vi "Load Test.vi"(8 "error in (no error)":errorcluster, 10 "Test Result 2":refnum<vi>, 11 "Data In":T1={"Message"="", "Homed?"=FALSE, "NextState"=enum."Timeout", "G.Load"=0.0, "G.Position"=0.0, "Load#"=0, "[G.Loads]"=[], "[TotalLoads]"=[], "[Errors]"=[], "ZeroWait"=0, "Results"=[], "DwellWait"=FALSE, "Test Result"=FALSE, "[CondyleLoads]"=[], "[Max]"=[], "[Min]"=[], "Valid String?"=FALSE, "ScanTime"=timestamp(0 s since 1904-01-01), "ScannedString"="", "LabelDevID"=0, "MfgDate"=timestamp(0 s since 1904-01-01), "[EEPROM Cmds]"=[], "[CalData]"=[], "[A/Ds]"=[], "[A/Dmax]"=[], "[A/Dmin]"=[], "BattMax"=0.0, "BattMin"=0.0, "DwellTime"=2000, "PendingDeviceType"="", "Zero G.load"=0.0, "GAINC Value"="", "Programming Step"=enum."Load EEPROM", "Front Panel Program?"=FALSE, "Final Program?"=FALSE, "PCB Score"=100, "AssyScore"=100, "Pass/Fail #"="", "Result String"="", "Programming Mode"=enum."Initial Program", "Angle Test Step"=enum."Initialize", "Accel Values"=[], "Shutdown Counter"=0, "V1"=0, "V2"=0, "V3"=0, "V4"=0, "EEPROM Data"=[], "Counter"=0, "Page#"=0, "Timer"=timestamp(0 s since 1904-01-01), "Use Mark10?"=FALSE, "Eng-Result#"=0, "DUT Serial #"=0, "Scroll Message?"=FALSE, "Clear Message"=FALSE, "Batt Test Step "=enum."Initialize", "RXTX Window Found?"=FALSE, "Shutdown First Call?"=FALSE, "A2 Delay (msec)"=500, "Support Script"={"Script #"="", "Script Revision"="", "[OEMs]"=[], "[[DeviceTypes]]"=[], "[[DeviceTypesVals]]"=[], "[[List of Errors]]"=[], "Default GAINC"="", "[[ASICtrims]]"=[], "ID For Echo"="", "Condyle A CalFactor"=100, "Condyle B CalFactor"=100, "[OEMs Prefix]"=[], "Packet ID 18"="", "[[Force Table Load Test]]"=[], "[[Force Table AccurTest]]"=[]}, "Serial Table"={"Serial File Path"=path "", "[[Serial Lookup Table]]"=[], "Serial Device Info"=[], "Valid Serial?"=FALSE}, "Target Information"={"Target Brand"="", "Target DeviceType"="", "Target Serial#"=100, "Target Lot#"=0, "Target DevID"=0, "Target Channel"=5}, "Operator"="", "COM Port"="", "Config Path"=path "", "Tx Array"=[], "DUT Parameters"={"Channel"=0, "DeviceID"=0, "Script Rev"=0, "Month"=0, "Day"=0, "Year"=0, "Lot#"=0, "V1"=0, "V2"=0, "V3"=0, "V4"=0, "MFG"=0, "Cal FactorA 10"=0, "Cal FactorB 10  "=0, "Cal FactorA 16"=0, "Cal FactorB 16"=0, "ASICtrim"=[], "TmpChan"=0, "GAINC"="", "Brand"="", "Device"="", "Serial #"=0, "Batt310"=0, "Batt 280"=0}, "FTS Main?"=FALSE, "Loading"={"[Forces]"=[], "[Dwell]"=[], "Loading Step"=enum."Initialize Test"}, "Software Version"="", "Correction Factor"="", "Second Load Test"=FALSE, "Acc Loads"=[], "Mark10 Config"={"H2S%"=[80.0, 85.0, 90.0, 95.0, 100.0], "H2S Speed"=[12.0, 8.0, 6.0, 4.0, 2.0], "H to S"=2.0, "Home Speed"=1.0, "LoadWin"=0.0, "Load Speed"=0.0, "PID"={"Kp"=0.04, "Kd"=0.005001, "Ki"=2.9999999999999923e-05}}, "Channels"={"Transceiver Ch"=5, "Operating Ch"=5, "Start Ch"=0}, "Channel EEPROM"=[], "Load Notes"=[], "Engr Log?"=FALSE, "Time"=[], "Program Retry"=FALSE, "Operator Channel"="", "Target Channel "="", "New Data Program"=FALSE, "NFHU Pass?"=FALSE, "Cycle Number"=0, "Cal Cycle#"=0, "[Avg G.Loads] "=[], "[Avg A/Ds] "=[], "Cal Retry?"=FALSE, "[Total A/Ds]  "=[], "Cycle Num LA"=0, "LA Cycle# "=0, "Shim Num"=0, "Shim#  "=0, "Angle Test?"=FALSE} {"Mark10 Config"."PID"."Ki" min=0.0 max=200.0 format="%.6f"; "Mark10 Config"."PID"."Kd" min=0.0 max=200.0 format="%.6f"; "Mark10 Config"."PID"."Kp" min=0.0 max=200.0 format="%.6f"; "DUT Parameters"."ASICtrim" format="%02x"}) -> (0 "error out":errorcluster, 1 "LoadSensors":dbl[](array[numeric]), 3 "State-machine Local Variables out":T1={"Message"="", "Homed?"=FALSE, "NextState"=enum."Timeout", "G.Load"=0.0, "G.Position"=0.0, "Load#"=0, "[G.Loads]"=[], "[TotalLoads]"=[], "[Errors]"=[], "ZeroWait"=0, "Results"=[], "DwellWait"=FALSE, "Test Result"=FALSE, "[CondyleLoads]"=[], "[Max]"=[], "[Min]"=[], "Valid String?"=FALSE, "ScanTime"=timestamp(0 s since 1904-01-01), "ScannedString"="", "LabelDevID"=0, "MfgDate"=timestamp(0 s since 1904-01-01), "[EEPROM Cmds]"=[], "[CalData]"=[], "[A/Ds]"=[], "[A/Dmax]"=[], "[A/Dmin]"=[], "BattMax"=0.0, "BattMin"=0.0, "DwellTime"=2000, "PendingDeviceType"="", "Zero G.load"=0.0, "GAINC Value"="", "Programming Step"=enum."Load EEPROM", "Front Panel Program?"=FALSE, "Final Program?"=FALSE, "PCB Score"=100, "AssyScore"=100, "Pass/Fail #"="", "Result String"="", "Programming Mode"=enum."Initial Program", "Angle Test Step"=enum."Initialize", "Accel Values"=[], "Shutdown Counter"=0, "V1"=0, "V2"=0, "V3"=0, "V4"=0, "EEPROM Data"=[], "Counter"=0, "Page#"=0, "Timer"=timestamp(0 s since 1904-01-01), "Use Mark10?"=FALSE, "Eng-Result#"=0, "DUT Serial #"=0, "Scroll Message?"=FALSE, "Clear Message"=FALSE, "Batt Test Step "=enum."Initialize", "RXTX Window Found?"=FALSE, "Shutdown First Call?"=FALSE, "A2 Delay (msec)"=500, "Support Script"={"Script #"="", "Script Revision"="", "[OEMs]"=[], "[[DeviceTypes]]"=[], "[[DeviceTypesVals]]"=[], "[[List of Errors]]"=[], "Default GAINC"="", "[[ASICtrims]]"=[], "ID For Echo"="", "Condyle A CalFactor"=100, "Condyle B CalFactor"=100, "[OEMs Prefix]"=[], "Packet ID 18"="", "[[Force Table Load Test]]"=[], "[[Force Table AccurTest]]"=[]}, "Serial Table"={"Serial File Path"=path "", "[[Serial Lookup Table]]"=[], "Serial Device Info"=[], "Valid Serial?"=FALSE}, "Target Information"={"Target Brand"="", "Target DeviceType"="", "Target Serial#"=100, "Target Lot#"=0, "Target DevID"=0, "Target Channel"=5}, "Operator"="", "COM Port"="", "Config Path"=path "", "Tx Array"=[], "DUT Parameters"={"Channel"=0, "DeviceID"=0, "Script Rev"=0, "Month"=0, "Day"=0, "Year"=0, "Lot#"=0, "V1"=0, "V2"=0, "V3"=0, "V4"=0, "MFG"=0, "Cal FactorA 10"=0, "Cal FactorB 10  "=0, "Cal FactorA 16"=0, "Cal FactorB 16"=0, "ASICtrim"=[], "TmpChan"=0, "GAINC"="", "Brand"="", "Device"="", "Serial #"=0, "Batt310"=0, "Batt 280"=0}, "FTS Main?"=FALSE, "Loading"={"[Forces]"=[], "[Dwell]"=[], "Loading Step"=enum."Initialize Test"}, "Software Version"="", "Correction Factor"="", "Second Load Test"=FALSE, "Acc Loads"=[], "Mark10 Config"={"H2S%"=[80.0, 85.0, 90.0, 95.0, 100.0], "H2S Speed"=[12.0, 8.0, 6.0, 4.0, 2.0], "H to S"=2.0, "Home Speed"=1.0, "LoadWin"=0.0, "Load Speed"=0.0, "PID"={"Kp"=0.04, "Kd"=0.005001, "Ki"=2.9999999999999923e-05}}, "Channels"={"Transceiver Ch"=5, "Operating Ch"=5, "Start Ch"=0}, "Channel EEPROM"=[], "Load Notes"=[], "Engr Log?"=FALSE, "Time"=[], "Program Retry"=FALSE, "Operator Channel"="", "Target Channel "="", "New Data Program"=FALSE, "NFHU Pass?"=FALSE, "Cycle Number"=0, "Cal Cycle#"=0, "[Avg G.Loads] "=[], "[Avg A/Ds] "=[], "Cal Retry?"=FALSE, "[Total A/Ds]  "=[], "Cycle Num LA"=0, "LA Cycle# "=0, "Shim Num"=0, "Shim#  "=0, "Angle Test?"=FALSE} {"Mark10 Config"."PID"."Ki" min=0.0 max=200.0 format="%.6f"; "Mark10 Config"."PID"."Kd" min=0.0 max=200.0 format="%.6f"; "Mark10 Config"."PID"."Kp" min=0.0 max=200.0 format="%.6f"; "DUT Parameters"."ASICtrim" format="%02x"}, 5 "Raw Data":u16[](array[numeric]))   [LabVIEW 2015]
uses:
  Controls/LocalVars.ctl
  Controls/Gen2 FT states.ctl
  Controls/Iniial Device Programming.ctl
  ProgramStageControl.ctl
  Controls/Batt Cap Steps.ctl
  Controls/Support Script.ctl
  Controls/Serial Table.ctl
  Controls/Device Information.ctl
  Controls/InfoPacket.ctl
  Controls/Loading.ctl
  Controls/Load Step.ctl
  Controls/Mark10 Config.ctl
  Controls/PID parameters.ctl
  Controls/Channels.ctl
  Controls/Mark10 states.ctl
  Controls/Gen2 FT Globals.vi
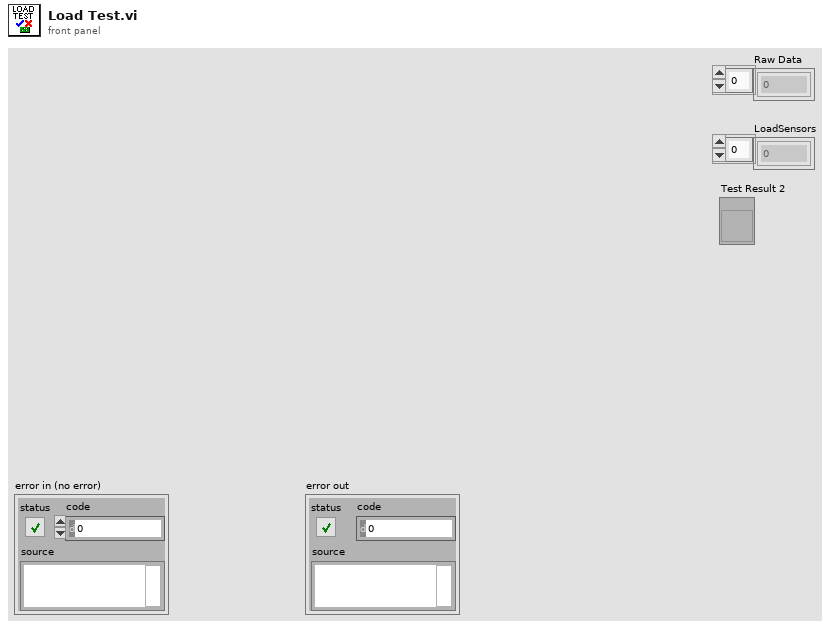
[diagram p1: front panel]
types:
  T1 = typedef "LocalVars.ctl" = cluster{"Message":string, "Homed?":bool, "NextState":T2, "G.Load":dbl, "G.Position":dbl, "Load#":i32, "[G.Loads]":dbl[], "[TotalLoads]":dbl[], "[Errors]":dbl[][], "ZeroWait":u32, "Results":dbl[], "DwellWait":bool, "Test Result":bool, "[CondyleLoads]":dbl[][], "[Max]":dbl[], "[Min]":dbl[], "Valid String?":bool, "ScanTime":timestamp, "ScannedString":string, "LabelDevID":u32, "MfgDate":timestamp, "[EEPROM Cmds]":u8[][], "[CalData]":u8[][], "[A/Ds]":dbl[][], "[A/Dmax]":dbl[], "[A/Dmin]":dbl[], "BattMax":dbl, "BattMin":dbl, "DwellTime":i32, "PendingDeviceType":string, "Zero G.load":dbl, "GAINC Value":string, "Programming Step":T3, "Front Panel Program?":bool, "Final Program?":bool, "PCB Score":i32, "AssyScore":i32, "Pass/Fail #":string, "Result String":string, "Programming Mode":T4, "Angle Test Step":enum16{"Initialize", "Get X", "Get Y", "Get Z", "Next Test"}, "Accel Values":dbl[][], "Shutdown Counter":u32, "V1":i32, "V2":i32, "V3":i32, "V4":i32, "EEPROM Data":i32[][], "Counter":i32, "Page#":i32, "Timer":timestamp, "Use Mark10?":bool, "Eng-Result#":u32, "DUT Serial #":i32, "Scroll Message?":bool, "Clear Message":bool, "Batt Test Step ":T5, "RXTX Window Found?":bool, "Shutdown First Call?":bool, "A2 Delay (msec)":i16, "Support Script":T6, "Serial Table":T7, "Target Information":T8, "Operator":string, "COM Port":string, "Config Path":path, "Tx Array":u8[], "DUT Parameters":T9, "FTS Main?":bool, "Loading":T10, "Software Version":string, "Correction Factor":string, "Second Load Test":bool, "Acc Loads":dbl[][], "Mark10 Config":T12, "Channels":T14, "Channel EEPROM":i32[][], "Load Notes":string[], "Engr Log?":bool, "Time":timestamp[], "Program Retry":bool, "Operator Channel":string, "Target Channel ":string, "New Data Program":bool, "NFHU Pass?":bool, "Cycle Number":i32, "Cal Cycle#":i32, "[Avg G.Loads] ":dbl[], "[Avg A/Ds] ":dbl[][], "Cal Retry?":bool, "[Total A/Ds]  ":dbl[][], "Cycle Num LA":i32, "LA Cycle# ":i32, "Shim Num":i32, "Shim#  ":i32, "Angle Test?":bool}
  T2 = typedef "Gen2 FT states.ctl" = enum16{"---------SETUP-------", "Initialization", "Read Support Data", "Initialize Mark-10", "Initialize Transceiver", "------UTILITIES------", "Change DUT Channel", "Find RxTx Window", "Reset Device", "Scan Channels", "Read Serial Lookup", "Shutdown Device", "ESTOP", "--------USER---------", "Timeout", "-----PROGRAM-----", "Program Device", "------MARK10--------", "Go Home", "MoveUp", "MoveDown", "Goto Load", "Goto Position", "Stop Motor", "---------TESTS--------", "Start Test", "Angle Test", "Load Test", "Load Accuracy Test", "Battery Test", "------RESULTS-------", "End Test", "Display Result", "--------EXIT--------", "Exit"}
  T3 = typedef "Iniial Device Programming.ctl" = enum16{"Load EEPROM", "Send First A1", "Send EEPROM", "Send A1", "Check EEPROM Echo", "Verify transmission", "Programming Successful", "Programming Failed"}
  T4 = typedef "ProgramStageControl.ctl" = enum16{"Initial Program", "GainC", "Scales"}
  T5 = typedef "Batt Cap Steps.ctl" = enum16{"Initialize", "Collect 2.8 Volts", "Collect 3.1 Volts", "Check Results"}
  T6 = typedef "Support Script.ctl" = cluster{"Script #":string, "Script Revision":string, "[OEMs]":string[], "[[DeviceTypes]]":string[][], "[[DeviceTypesVals]]":u16[][], "[[List of Errors]]":string[][], "Default GAINC":string, "[[ASICtrims]]":u8[][], "ID For Echo":string, "Condyle A CalFactor":i32, "Condyle B CalFactor":i32, "[OEMs Prefix]":string[], "Packet ID 18":string, "[[Force Table Load Test]]":dbl[][], "[[Force Table AccurTest]]":dbl[][]}
  T7 = typedef "Serial Table.ctl" = cluster{"Serial File Path":path, "[[Serial Lookup Table]]":string[][], "Serial Device Info":string[], "Valid Serial?":bool}
  T8 = typedef "Device Information.ctl" = cluster{"Target Brand":string, "Target DeviceType":string, "Target Serial#":i32, "Target Lot#":u32, "Target DevID":u32, "Target Channel":u8}
  T9 = typedef "InfoPacket.ctl" = cluster{"Channel":u8, "DeviceID":u32, "Script Rev":u8, "Month":u8, "Day":u8, "Year":u8, "Lot#":u32, "V1":u16, "V2":u16, "V3":u16, "V4":u16, "MFG":u8, "Cal FactorA 10":u8, "Cal FactorB 10  ":u8, "Cal FactorA 16":u8, "Cal FactorB 16":u8, "ASICtrim":u8[], "TmpChan":u8, "GAINC":string, "Brand":string, "Device":string, "Serial #":u64, "Batt310":u16, "Batt 280":u16}
  T10 = typedef "Loading.ctl" = cluster{"[Forces]":dbl[], "[Dwell]":dbl[], "Loading Step":T11}
  T11 = typedef "Load Step.ctl" = enum16{"Initialize Test", "Go Home", "Detect Dev Surface", "Wait to zero Device", "Zero Device", "Do Test", "Test Result"}
  T12 = typedef "Mark10 Config.ctl" = cluster{"H2S%":dbl[], "H2S Speed":dbl[], "H to S":dbl, "Home Speed":dbl, "LoadWin":dbl, "Load Speed":dbl, "PID":T13}
  T13 = typedef "PID parameters.ctl" = cluster{"Kp":dbl, "Kd":dbl, "Ki":dbl}
  T14 = typedef "Channels.ctl" = cluster{"Transceiver Ch":u8, "Operating Ch":u8, "Start Ch":u8}
  T15 = typedef "DeviceInfo.ctl" = cluster{"DevInfo":T9, "Mfg Date":timestamp, "[CalData]":u8[][], "[DevData]":u8[], "GotCal":bool, "CustomCal?":bool, "Packet#":i32}
  T16 = typedef "Mark10 states.ctl" = enum16{"Initialize", "Go Home", "Move Up", "Move Down", "Stop @ Load", "Read Status", "Goto Position", "Goto Device Surface", "Stop Motor", "Shutdown", "Exit"}
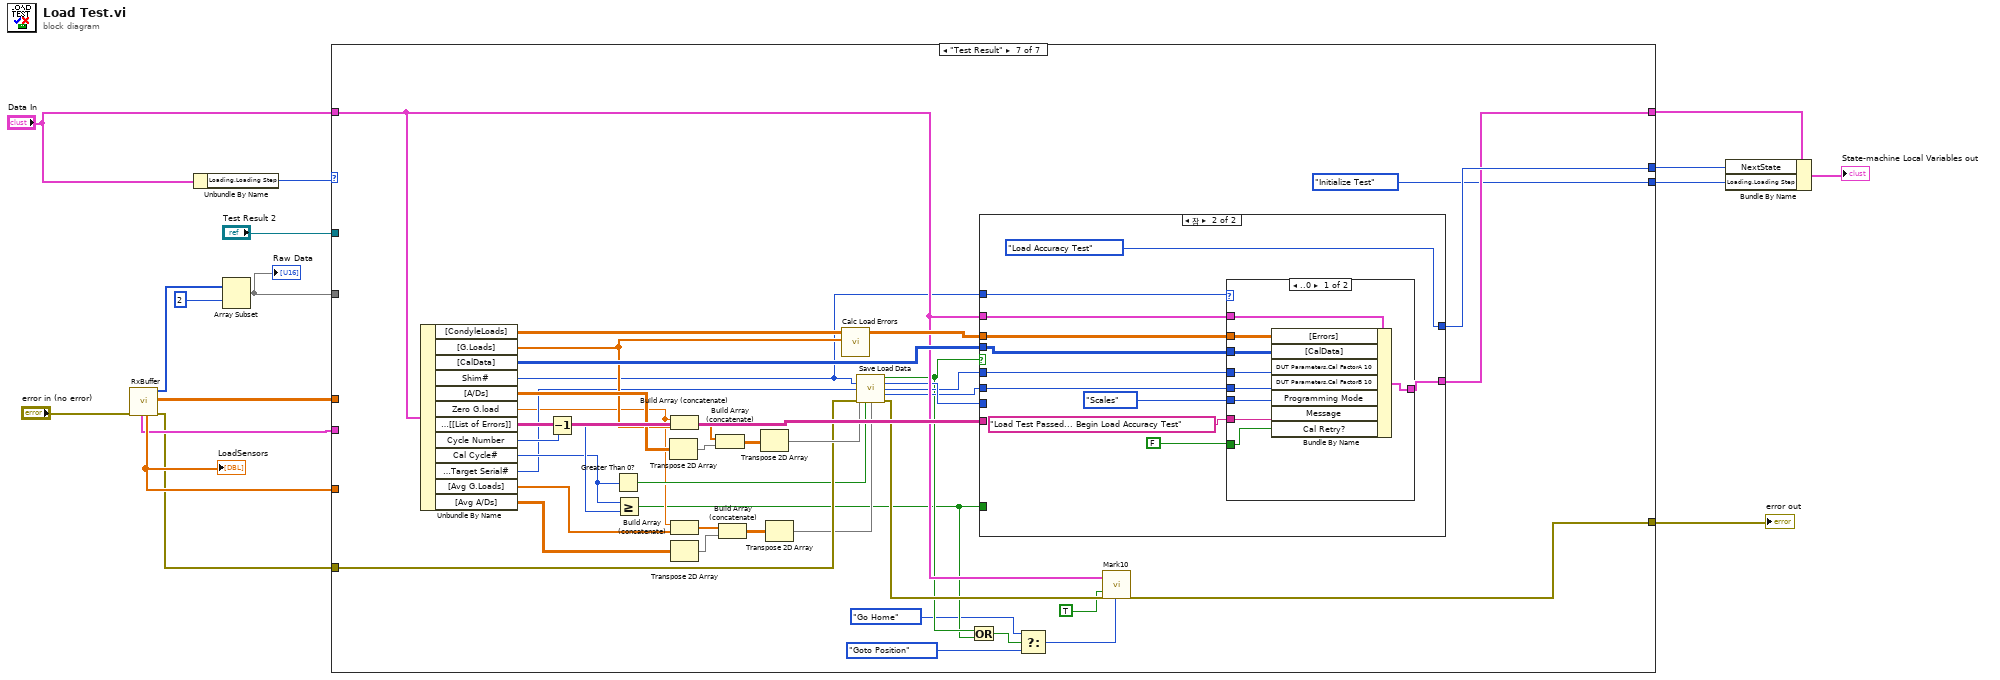
[diagram p0: block diagram]
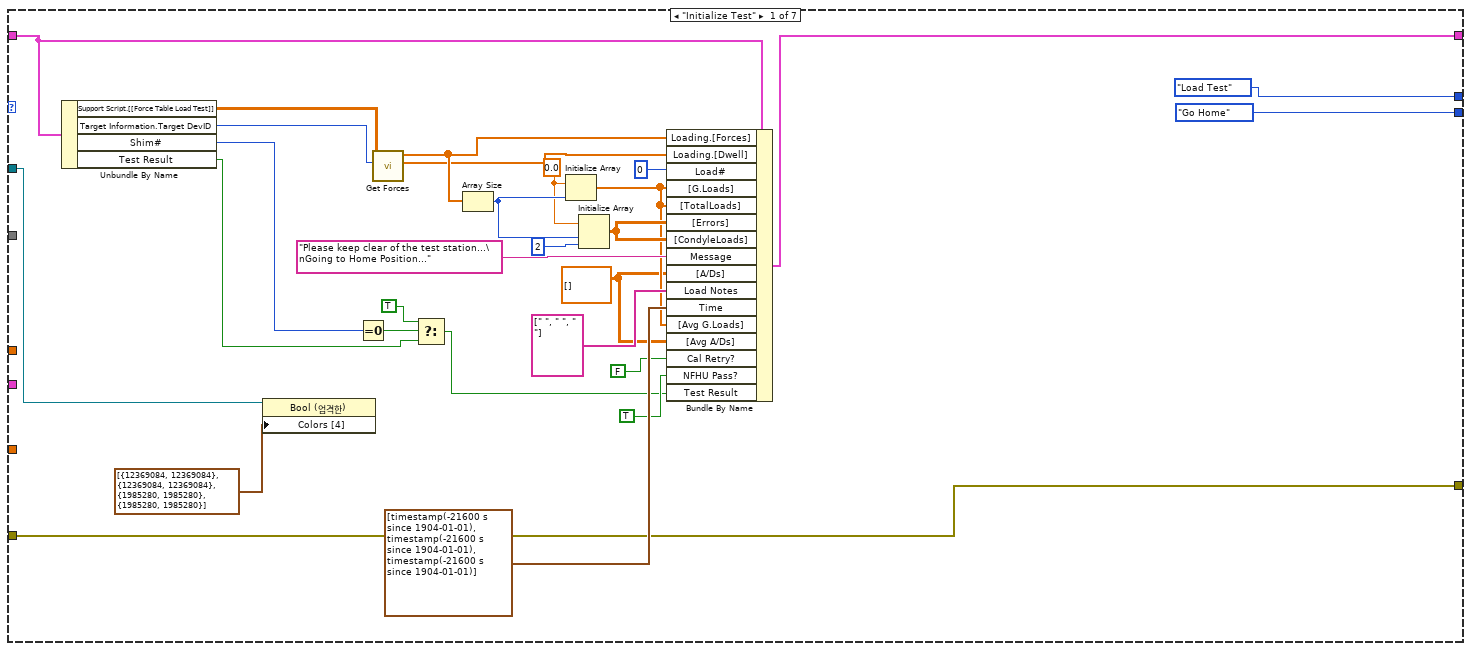
[diagram p2: hidden frame]
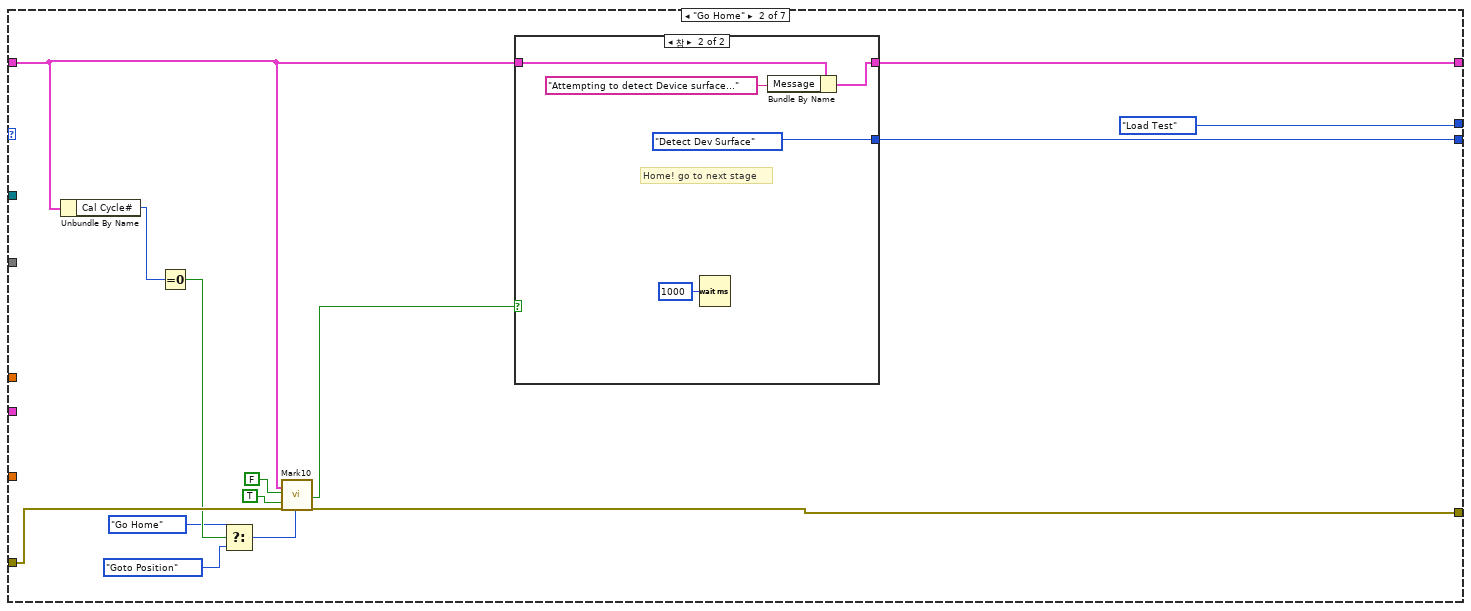
[diagram p3: hidden frame]
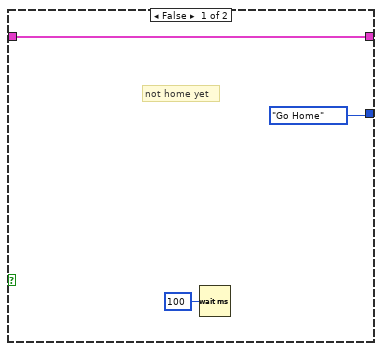
[diagram p4: hidden frame]
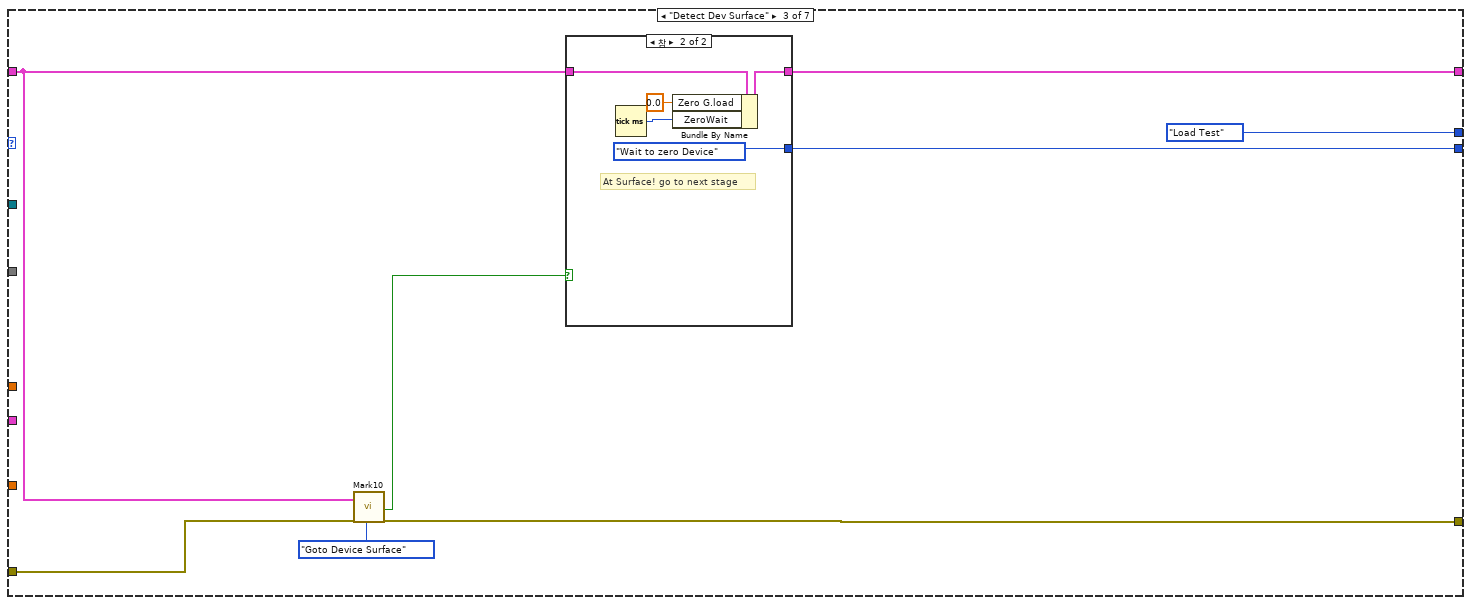
[diagram p5: hidden frame]
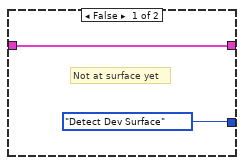
[diagram p6: hidden frame]
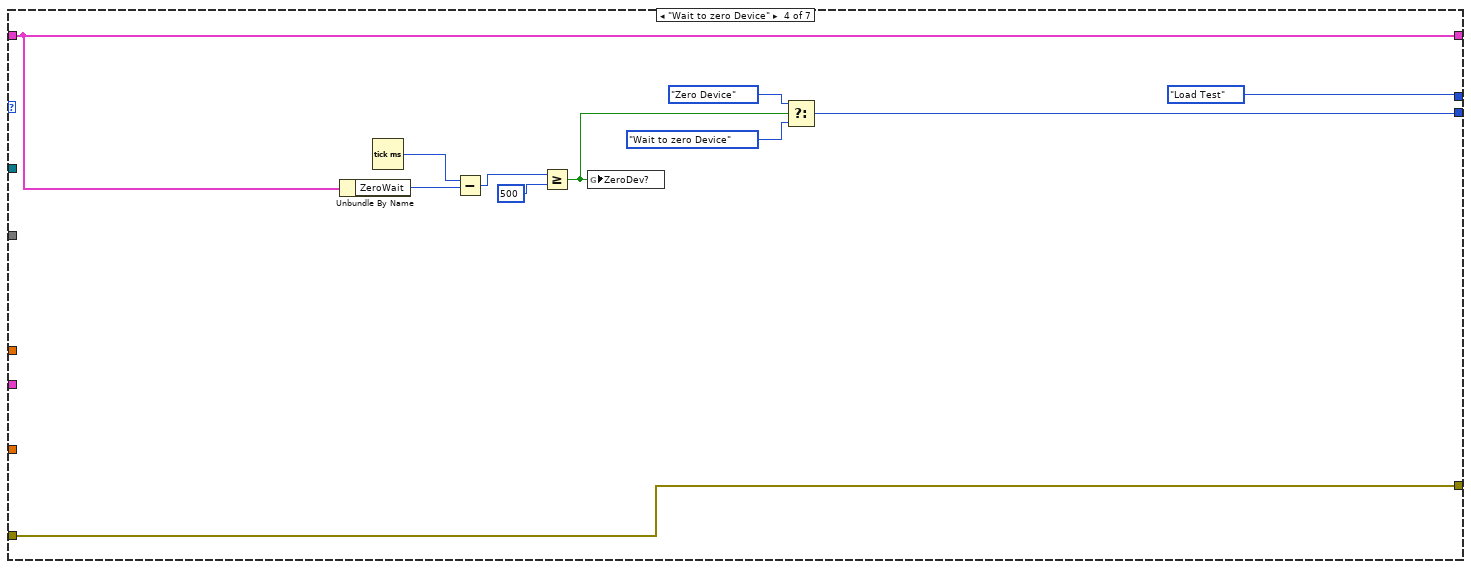
[diagram p7: hidden frame]
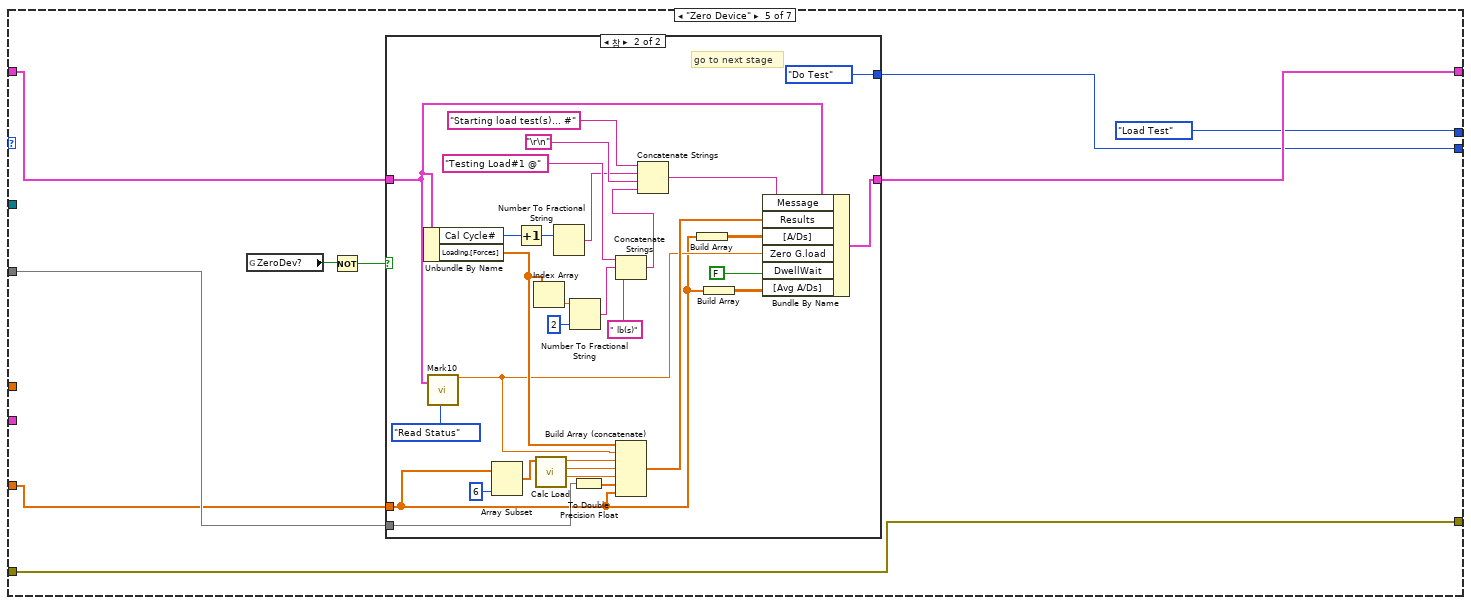
[diagram p8: hidden frame]
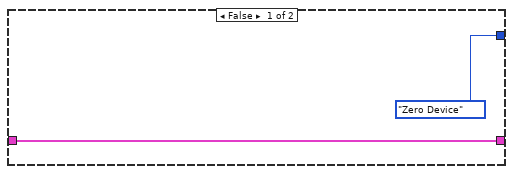
[diagram p9: hidden frame]
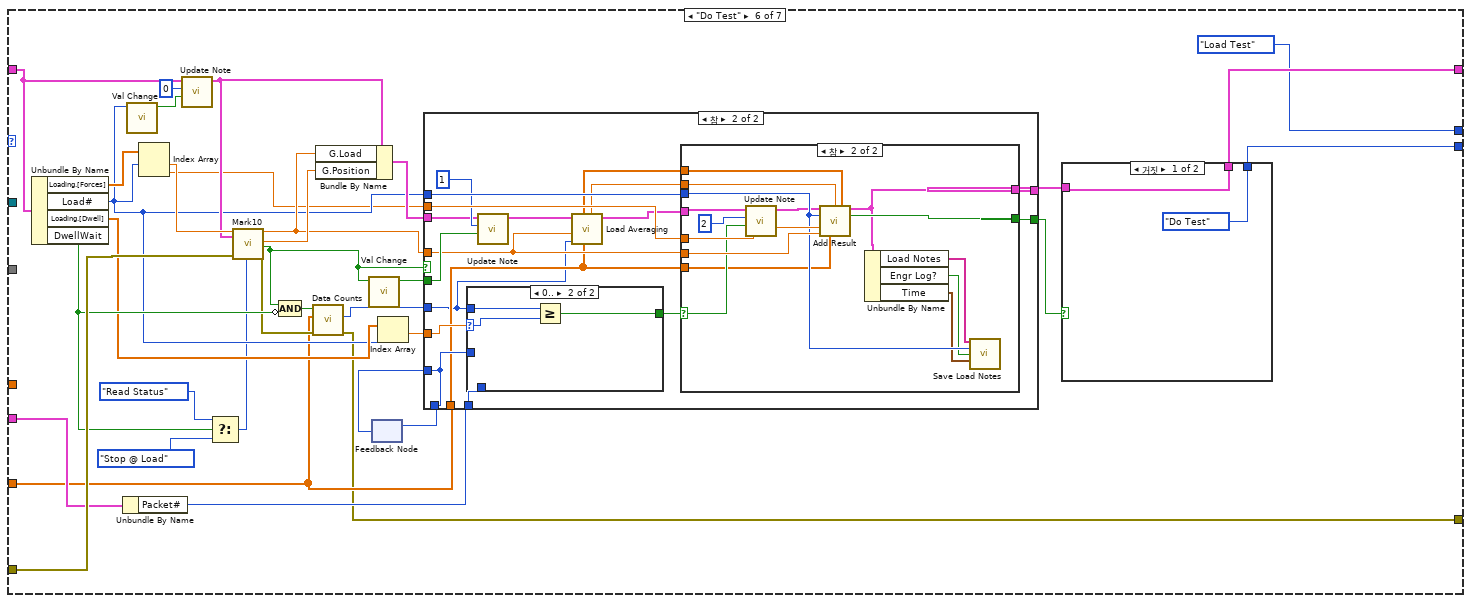
[diagram p10: hidden frame]
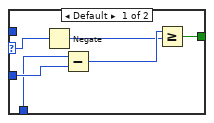
[diagram p12: hidden frame]
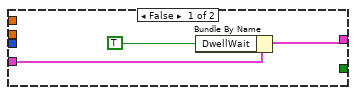
[diagram p13: hidden frame]
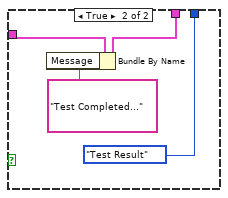
[diagram p14: hidden frame]
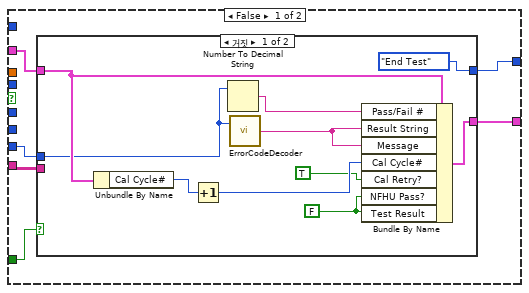
[diagram p15: hidden frame]
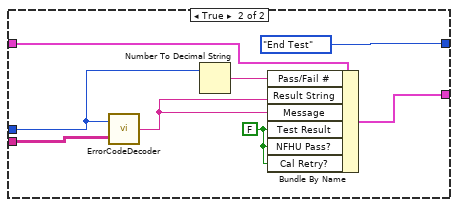
[diagram p16: hidden frame]
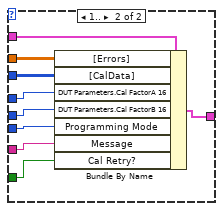
[diagram p17: hidden frame]
diagram:
  n1 = call "RxBuffer.vi"("error in (no error)"="error in (no error)") -> ("DeviceParameters"=w11:T15, "LoadSensors"=w12:dbl[], "RxData Out"=w9:u16[], "CalData"=w13:dbl[][], "error out"=w8:errorcluster)  [unwired: 7 in, 7 out]
  "LoadSensors" <- w12
  n2 = Unbundle By Name("Data In") -> ("Loading.Loading Step"=w4:T11)
  n3 = Array Subset(array=w9, index=2) -> (w14:u16[])  [unwired: 1 in]
  "Raw Data" <- w14
  n4 = case shown="\"Test Result\"" w4 {
    tunnel: [Load_Step."Go Home" ("Load Step") w53 w67 w82 w93 w149 Load_Step."Initialize Test" ("Load Step")] -> w3
    tunnel: "Data In" -> [w43 w51 w68 w91 w101 w146 w254]
    tunnel: [w44 w56 w72 w91 w100 w166 w253] -> w5
    tunnel: [w22 w57 w73 w92 w98 w134 w259] -> w6
    tunnel: w8 -> [w22 w58 w74 w92 w98 w167 w245]
    tunnel: w12 -> [_ _ _ _ w96 w136 _]
    tunnel: w14 -> [_ _ _ _ w97 _ _]
    tunnel: w11 -> [_ _ _ _ _ w140 _]
    tunnel: w13 -> [_ _ _ _ _ _ _]
    tunnel: [Gen2_FT_states."Load Test" ("NextState") Gen2_FT_states."Load Test" ("NextState") Gen2_FT_states."Load Test" ("NextState") Gen2_FT_states."Load Test" ("NextState") Gen2_FT_states."Load Test" ("NextState") Gen2_FT_states."Load Test" ("NextState") w255] -> w16
    tunnel: "Test Result 2" -> [w26 _ _ _ _ _ _]
    frame "Initialize Test" {
      w27 = dbl[][] [] ("[A/Ds]")
      w40 = 0.0 ("element")
      n5 = Unbundle By Name(w43) -> ("Support Script.[[Force Table Load Test]]"=w34:dbl[][], "Target Information.Target DevID"=w33:u32, "Shim#"=w21:i32, "Test Result"=w18:bool)
      n6 = property class="Bool (엄격한)"(reference=w26, "Colors [4]"=cluster{u32, u32}[] [{12369084, 12369084}, {12369084, 12369084}, {1985280, 1985280}, {1985280, 1985280}]) -> ()  [unwired: 1 in, 2 out]
      n7 = Equal To 0?(x=w21) -> (x = 0?=w20:bool)
      n8 = call "Get Forces.vi"("Device ID"=w33, "Force Table"=w34) -> ("Dwell"=w31:dbl[], "Forces"=w32:dbl[])  [unwired: 8 in]
      n9 = Select(t=TRUE, s=w20, f=w18) -> (s? t:f=w17:bool)
      n10 = Array Size(array=w32) -> (size(s)=w41:i32)
      n11 = Initialize Array(w40, w41) -> (w28:dbl[])
      n12 = Initialize Array(w40, w41, 2 ("dimension size")) -> (w38:dbl[][])
      n13 = Bundle By Name(cluster=w43, "Loading.[Forces]"=w32, "Loading.[Dwell]"=w31, "Load#"=0, "[G.Loads]"=w28, "[TotalLoads]"=w28, "[Errors]"=w38, "[CondyleLoads]"=w38, "Message"="Please keep clear of the test station...\nGoing to Home Position...", "[A/Ds]"=w27, "Load Notes"=string[] [" ", " ", " "], "Time"=timestamp[] [timestamp(-21600 s since 1904-01-01), timestamp(-21600 s since 1904-01-01), timestamp(-21600 s since 1904-01-01)], "[Avg G.Loads]"=w28, "[Avg A/Ds]"=w27, "Cal Retry?"=FALSE, "NFHU Pass?"=TRUE, "Test Result"=w17) -> (w44:T1)
    }
    frame "Go Home" {
      n14 = Unbundle By Name(w51) -> ("Cal Cycle#"=w50:i32)
      n15 = Equal To 0?(x=w50) -> (x = 0?=w49:bool)
      n16 = Select(t=Mark10_states."Go Home" ("Action"), s=w49, f=Mark10_states."Goto Position" ("Action")) -> (s? t:f=w46:T16)
      n17 = call "Mark10.vi"("Data In"=w51, "Stop?"=FALSE, "Accuracy \nTest?"=TRUE ("Stop?"), "error in (no error)"=w58, "Action"=w46) -> ("Done?"=w55:bool, "error out"=w57:errorcluster)  [unwired: 10 in, 3 out]
      n18 = case shown="참" w55 {
        tunnel: w51 -> [w61 w65]
        tunnel: [w61 w66] -> w56
        tunnel: [Load_Step."Go Home" ("Load Step") Load_Step."Detect Dev Surface" ("Load Step")] -> w53
        frame False {
          # "not home yet"
          n19 = Wait (ms)(milliseconds to wait=u32 100) -> ()  [unwired: 1 out]
        }
        frame True {
          # "Home! go to next stage"
          n20 = Wait (ms)(milliseconds to wait=u32 1000) -> ()  [unwired: 1 out]
          n21 = Bundle By Name(cluster=w65, "Message"="Attempting to detect Device surface...") -> (w66:T1)
        }
      }
    }
    frame "Detect Dev Surface" {
      n22 = call "Mark10.vi"("Data In"=w68, "error in (no error)"=w74, "Action"=Mark10_states."Goto Device Surface") -> ("Done?"=w71:bool, "error out"=w73:errorcluster)  [unwired: 12 in, 3 out]
      n23 = case shown="참" w71 {
        tunnel: w68 -> [w76 w80]
        tunnel: [w76 w81] -> w72
        tunnel: [Load_Step."Detect Dev Surface" ("Load Step") Load_Step."Wait to zero Device" ("Load Step")] -> w67
        frame False {
          # "Not at surface yet"
        }
        frame True {
          # "At Surface! go to next stage"
          n24 = Tick Count (ms)() -> (millisecond timer value=w78:u32)
          n25 = Bundle By Name(cluster=w80, "Zero G.load"=0.0, "ZeroWait"=w78) -> (w81:T1)
        }
      }
    }
    frame "Wait to zero Device" {
      n26 = Unbundle By Name(w91) -> ("ZeroWait"=w89:u32)
      n27 = Tick Count (ms)() -> (millisecond timer value=w90:u32)
      n28 = Subtract(x=w90, y=w89) -> (x-y=w88:u32)
      n29 = Greater Or Equal?(x=w88, y=u32 500) -> (x >= y?=w85:bool)
      n30 = global write "Gen2 FT Globals.vi" "ZeroDev?"(w85) -> ()
      n31 = Select(t=Load_Step."Zero Device" ("Load Step"), s=w85, f=Load_Step."Wait to zero Device" ("Load Step")) -> (s? t:f=w82:T11)
    }
    frame "Zero Device" {
      n32 = global read "Gen2 FT Globals.vi" "ZeroDev?"() -> (w99:bool)
      n33 = Not(x=w99) -> (.not. x?=w95:bool)
      n34 = case shown="참" w95 {
        tunnel: w101 -> [w103 w111]
        tunnel: [w103 w133] -> w100
        tunnel: w96 -> [_ w105]
        tunnel: w97 -> [_ w117]
        tunnel: [Load_Step."Zero Device" ("Load Step") Load_Step."Do Test" ("Load Step")] -> w93
        frame False {
        }
        frame True {
          # "go to next stage"
          n35 = Unbundle By Name(w111) -> ("Cal Cycle#"=w109:i32, "Loading.[Forces]"=w124:dbl[])
          n36 = call "Mark10.vi"("Data In"=w111, "Action"=Mark10_states."Read Status") -> ("Live Load"=w114:dbl)  [unwired: 13 in, 4 out]
          n37 = Array Subset(array=w105, length=6) -> (w121:dbl[])  [unwired: 1 in]
          n38 = Increment(x=w109) -> (x+1=w108:i32)
          n39 = Index Array(array=w124) -> (element=w125:dbl)  [unwired: 1 in]
          n40 = call "Calc Load.vi"("[A/D]"=w121) -> ("Condyle B Load"=w118:dbl, "Condyle A Load"=w119:dbl, "Total Load"=w120:dbl)  [unwired: 7 in, 1 out]
          n41 = Number To Fractional String(number=w108) -> (F-format string=w106:string)  [unwired: 3 in]
          n42 = Number To Fractional String(number=w125, precision (6)=i16 2) -> (F-format string=w130:string)  [unwired: 2 in]
          n43 = To Double Precision Float(number=w117) -> (double precision float=w116:dbl[])
          n44 = Concatenate Strings("Testing Load#1 @" ("Message"), w130, " lb(s)" ("Message")) -> (w126:string)
          n45 = Build Array (concatenate)(w124, w114, w120, w119, w118, w116, w105) -> (w123:dbl[])
          n46 = Concatenate Strings("Starting load test(s)... #" ("Message"), w106, "\r\n", w126) -> (w128:string)
          n47 = Build Array(w105) -> (w112:dbl[][])
          n48 = Build Array(w105) -> (w104:dbl[][])
          n49 = Bundle By Name(cluster=w111, "Message"=w128, "Results"=w123, "[A/Ds]"=w112, "Zero G.load"=w114, "DwellWait"=FALSE, "[Avg A/Ds]"=w104) -> (w133:T1)
        }
      }
    }
    frame "Do Test" {
      n50 = Unbundle By Name(w146) -> ("Loading.[Forces]"=w165:dbl[], "Load#"=w144:i32, "Loading.[Dwell]"=w152:dbl[], "DwellWait"=w156:bool)
      n51 = Unbundle By Name(w140) -> ("Packet#"=w155:i32)
      n52 = call "Val Change.vi"("data"=w144) -> ("Boolean"=w147:bool)  [unwired: 10 in]
      n53 = Index Array(array=w165, index #1=w144) -> (element #1=w160:dbl, element #2=w141:dbl)  [unwired: 1 in]
      n54 = call "Update Note.vi"("Update"=w147, "index"=0, "Data In in"=w146) -> ("Data In out"=w145:T1)  [unwired: 8 in]
      n55 = Select(t=Mark10_states."Read Status" ("Action"), s=w156, f=Mark10_states."Stop @ Load" ("Action")) -> (s? t:f=w139:T16)
      n56 = call "Mark10.vi"("Requested Load"=w160, "Data In"=w145, "error in (no error)"=w167, "Action"=w139) -> ("Live Load"=w161:dbl, "Live Position"=w162:dbl, "Done?"=w143:bool, "error out"=w137:errorcluster)  [unwired: 11 in, 1 out]
      n57 = Compound Arithmetic op=AND(w143, invert w156) -> (w138:bool)
      n58 = call "Data Counts.vi"("error in (no error)"=w137, "Data"=w136, "Initialize"=w138) -> ("error out"=w134:errorcluster, "Data Points"=w135:i32)  [unwired: 7 in]
      n59 = Bundle By Name(cluster=w145, "G.Load"=w161, "G.Position"=w162) -> (w163:T1)
      n60 = call "Val Change.vi"("data"=w143) -> ("Boolean"=w142:bool)  [unwired: 10 in]
      n61 = feedback #1() -> (w153:i32)  [unwired: 1 in]
      n62 = Index Array(array=w152, index=w144) -> (element=w151:dbl)
      n63 = case shown="참" w143 {
        tunnel: w163 -> [w169 w177]
        tunnel: w144 -> [_ w185]
        tunnel: [_ w187] -> w164
        tunnel: w161 -> [_ w176]
        tunnel: w141 -> [_ w186]
        tunnel: w135 -> [_ w170]
        tunnel: [w169 w184] -> w159
        tunnel: w151 -> [_ w181]
        tunnel: w155 -> [w168 w180]
        tunnel: [w168 w182] -> w154
        tunnel: w153 -> [_ w182]
        tunnel: w142 -> [_ w178]
        tunnel: w136 -> [_ w173]
        frame False {
        }
        frame True {
          n64 = case shown="0.." w181 {
            selector: w181 -> [w189 w194]
            tunnel: w170 -> [_ w196]
            tunnel: [w191 w195] -> w183
            tunnel: w182 -> [w193 _]
            tunnel: w180 -> [w190 _]
            frame Default {
              n65 = Negate(x=w189) -> (-x=w188:i32)
              n66 = Subtract(x=w190, y=w193) -> (x-y=w192:i32)
              n67 = Greater Or Equal?(x=w192, y=w188) -> (x >= y?=w191:bool)
            }
            frame 0.. {
              n68 = Greater Or Equal?(x=w196, y=w194) -> (x >= y?=w195:bool)
            }
          }
          n69 = call "Update Note.vi"("Update"=w178, "index"=1, "Data In in"=w177) -> ("Data In out"=w175:T1)  [unwired: 8 in]
          n70 = call "Load Averaging.vi"("Load Sensors"=w173, "Data Points"=w170, "Gauge Load"=w176, "Data In in"=w175) -> ("Data In out"=w174:T1, "Average G Load"=w172:dbl, "Average Load Sensors"=w171:dbl[])  [unwired: 4 in, 1 out]
          n71 = case shown="참" w183 {
            selector: w183 -> [_ w205]
            tunnel: w174 -> [w199 w208]
            tunnel: [w198 w211] -> w184
            tunnel: [_ w214] -> w187
            tunnel: w186 -> [_ w212]
            tunnel: w185 -> [_ w209]
            tunnel: w176 -> [_ w213]
            tunnel: w173 -> [_ w202]
            tunnel: w172 -> [_ w201]
            tunnel: w171 -> [_ w200]
            frame False {
              n72 = Bundle By Name(cluster=w199, "DwellWait"=TRUE) -> (w198:T1)
            }
            frame True {
              n73 = call "Update Note.vi"("Update"=w205, "index"=2, "Data In in"=w208) -> ("Data In out"=w207:T1)  [unwired: 8 in]
              n74 = call "Add Result.vi"("State-machine Local Variables in"=w207, "Avg Live Load"=w201, "[Avg LoadSensors]"=w200, "Load#"=w209, "SetLoad"=w212, "Live Load"=w213, "[LoadSensors]"=w202) -> ("State-machine Local Variables out"=w211:T1, "Done"=w214:bool)  [unwired: 7 in]
              n75 = Unbundle By Name(w211) -> ("Load Notes"=w210:string[], "Engr Log?"=w203:bool, "Time"=w204:timestamp[])
              n76 = call "Save Load Notes.vi"("Load Notes"=w210, "Load#"=w209, "Log?"=w203, "Time"=w204) -> ()  [unwired: 11 in, 1 out]
            }
          }
        }
      }
      n77 = feedback-in #1(w154) -> ()
      n78 = case shown="거짓" w164 {
        tunnel: w159 -> [w216 w220]
        tunnel: [w216 w219] -> w166
        tunnel: [Load_Step."Do Test" ("Load Step") Load_Step."Test Result" ("Load Step")] -> w149
        frame False {
        }
        frame True {
          n79 = Bundle By Name(cluster=w220, "Message"="Test Completed...") -> (w219:T1)
        }
      }
    }
    frame "Test Result" {
      n80 = Unbundle By Name(w254) -> ("[CondyleLoads]"=w260:dbl[][], "[G.Loads]"=w247:dbl[], "[CalData]"=w256:u8[][], "Shim#"=w221:i32, "[A/Ds]"=w248:dbl[][], "Zero G.load"=w235:dbl, "Support Script.[[List of Errors]]"=w258:string[][], "Cycle Number"=w240:i32, "Cal Cycle#"=w238:i32, "Target Information.Target Serial#"=w236:i32, "[Avg G.Loads]"=w234:dbl[], "[Avg A/Ds]"=w233:dbl[][])
      n81 = Decrement(x=w240) -> (x-1=w239:i32)
      n82 = Greater Than 0?(x=w238) -> (x > 0?=w237:bool)
      n83 = Greater Or Equal?(x=w238, y=w239) -> (x >= y?=w227:bool)
      n84 = Transpose 2D Array(2D array=w248) -> (transposed array=w251:dbl[][])
      n85 = Build Array (concatenate)(w235, w247) -> (w249:dbl[])
      n86 = Build Array (concatenate)(w235, w234) -> (w232:dbl[])
      n87 = Transpose 2D Array(2D array=w233) -> (transposed array=w231:dbl[][])
      n88 = Build Array (concatenate)(w249, w251) -> (w250:dbl[][])
      n89 = Build Array (concatenate)(w232, w231) -> (w230:dbl[][])
      n90 = Transpose 2D Array(2D array=w250) -> (transposed array=w246:dbl[][])
      n91 = Transpose 2D Array(2D array=w230) -> (transposed array=w229:dbl[][])
      n92 = call "Calc Load Errors.vi"("[G.Loads]"=w247, "[CondyleLoads]"=w260) -> ("Load Errors"=w257:dbl[][])  [unwired: 9 in]
      n93 = call "Save Load Data.vi"("[A/D Input]"=w246, "Shim #"=w221, "Eng-Result #"=w236, "error in (no error)"=w245, "Re Create New Engr Results? (F)"=w237, "[Avg A/D Input]"=w229) -> ("Pass?"=w228:bool, "Error Code"=w243:i32, "ScaleA"=w242:i32, "ScaleB"=w241:i32, "error out"=w244:errorcluster)  [unwired: 5 in]
      n94 = Or(x=w228, y=w227) -> (x .or. y?=w226:bool)
      n95 = case shown="참" w228 {
        tunnel: w243 -> [w265 _]
        tunnel: w258 -> [w266 _]
        tunnel: w257 -> [_ w295]
        tunnel: w256 -> [_ w293]
        tunnel: w242 -> [_ w292]
        tunnel: w241 -> [_ w291]
        tunnel: [w264 Gen2_FT_states."Load Accuracy Test" ("NextState")] -> w255
        tunnel: w254 -> [w263 w288]
        tunnel: [w262 w287] -> w253
        tunnel: w227 -> [w261 _]
        tunnel: w221 -> [_ w285]
        frame False {
          n96 = case shown="거짓" w261 {
            tunnel: w266 -> [_ w283]
            tunnel: w265 -> [w271 w282]
            tunnel: [Gen2_FT_states."End Test" ("NextState") Gen2_FT_states."End Test" ("NextState")] -> w264
            tunnel: w263 -> [w274 w279]
            tunnel: [w273 w278] -> w262
            frame False {
              w267 = FALSE
              n97 = Unbundle By Name(w274) -> ("Cal Cycle#"=w275:i32)
              n98 = Increment(x=w275) -> (x+1=w272:i32)
              n99 = Number To Decimal String(number=w271) -> (decimal integer string=w270:string)  [unwired: 1 in]
              n100 = call "ErrorCodeDecoder.vi"("FTS Error Code In"=w271) -> ("Error Message"=w268:string)  [unwired: 1 in]
              n101 = Bundle By Name(cluster=w274, "Pass/Fail #"=w270, "Result String"=w268, "Message"=w268, "Cal Cycle#"=w272, "Cal Retry?"=TRUE, "NFHU Pass?"=w267, "Test Result"=w267) -> (w273:T1)
            }
            frame True {
              w277 = FALSE ("Test Result")
              n102 = call "ErrorCodeDecoder.vi"("array"=w283, "FTS Error Code In"=w282) -> ("Error Message"=w281:string)
              n103 = Number To Decimal String(number=w282) -> (decimal integer string=w284:string)  [unwired: 1 in]
              n104 = Bundle By Name(cluster=w279, "Pass/Fail #"=w284, "Result String"=w281, "Message"=w281, "Test Result"=w277, "NFHU Pass?"=w277, "Cal Retry?"=w277) -> (w278:T1)
            }
          }
        }
        frame True {
          n105 = case shown="..0" w285 {
            tunnel: w295 -> [w304 w307]
            tunnel: ProgramStageControl."Scales" ("Program Stage") -> [w303 w311]
            tunnel: w293 -> [w302 w308]
            tunnel: w292 -> [w301 w306]
            tunnel: w291 -> [w300 w305]
            tunnel: "Load Test Passed... Begin Load Accuracy Test" ("Message") -> [w299 w310]
            tunnel: w288 -> [w298 w313]
            tunnel: [w297 w312] -> w287
            tunnel: FALSE -> [w296 w309]
            frame ..0 {
              n106 = Bundle By Name(cluster=w298, "[Errors]"=w304, "[CalData]"=w302, "DUT Parameters.Cal FactorA 10"=w301, "DUT Parameters.Cal FactorB 10"=w300, "Programming Mode"=w303, "Message"=w299, "Cal Retry?"=w296) -> (w297:T1)
            }
            frame 1.. {
              n107 = Bundle By Name(cluster=w313, "[Errors]"=w307, "[CalData]"=w308, "DUT Parameters.Cal FactorA 16"=w306, "DUT Parameters.Cal FactorB 16"=w305, "Programming Mode"=w311, "Message"=w310, "Cal Retry?"=w309) -> (w312:T1)
            }
          }
        }
      }
      n108 = Select(t=Mark10_states."Go Home" ("Action"), s=w226, f=Mark10_states."Goto Position" ("Action")) -> (s? t:f=w224:T16)
      n109 = call "Mark10.vi"("Data In"=w254, "Accuracy \nTest?"=TRUE, "error in (no error)"=w244, "Action"=w224) -> ("error out"=w259:errorcluster)  [unwired: 11 in, 4 out]
    }
  }
  "error out" <- w6
  n110 = Bundle By Name(cluster=w5, "NextState"=w16, "Loading.Loading Step"=w3) -> (→"State-machine Local Variables out":T1)
